vi "Serialize.vi"(8 "error in":errorcluster, 9 "OwningElement in":refnum<k20>, 10 "Document in":refnum<k20>, 11 "CustomDataType in":refnum<class "CustomData.lvclass">) -> (0 "error out":errorcluster, 1 "OwningElement out":refnum<k20>, 2 "Document out":refnum<k20>, 3 "CustomDataType out":refnum<class "CustomData.lvclass">)   [LabVIEW 2021, in "ProligentXMLGenerator.lvlib" / "CustomData.lvclass"]
uses:
  CustomData.lvclass
  CustomData.lvclass/CustomData.ctl
  Base/DOMSupport/DOMSupport.lvlib
  <vilib>/xml/NI_XML.lvlib
  <vilib>/xml/Close Reference(Node).vi
  CustomElement/CustomElement.lvclass
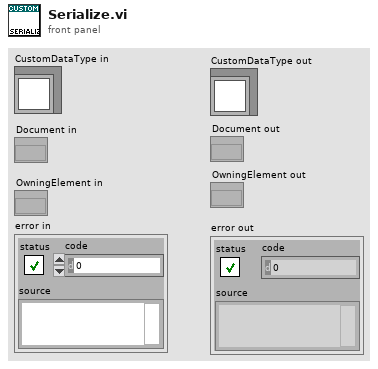
[diagram p1: front panel]
types:
  T1 = typedef "ProligentXMLGenerator.lvlib/CustomData.lvclass/Data.ctl" = cluster{"Name":string, "CustomElements":refnum<class "CustomElement.lvclass">[]}
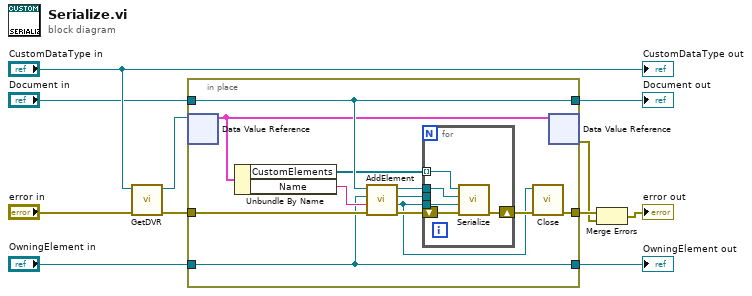
[diagram p0: block diagram]
diagram:
  n1 = call "GetDVR.vi"("error in"="error in", "CustomDataType"="CustomDataType in") -> ("error out"=w3:errorcluster, "DVRReference"=w2:refnum<data-value>)  [unwired: 8 in]
  n2 = in-place "In Place Element Structure" {
    in-place-border: [w21] -> w4
    in-place-border: "Document in" -> [w20]
    in-place-border: w3 -> [w23]
    in-place-border: "OwningElement in" -> [w19]
    in-place-border: [w20] -> w6
    in-place-border: [w19] -> w5
    n3 = in-place-dvr #1(w2) -> (w18:T1)  [unwired: 1 out]
    n4 = Unbundle By Name(w18) -> ("CustomElements"=w15:refnum<class "CustomElement.lvclass">[], "Name"=w22:string)
    n5 = call "AddElement.vi"("error in"=w23, "Name"=w22, "OwningElement in"=w19, "Document in"=w20) -> ("error out"=w17:errorcluster, "NewElement"=w13:refnum<k20>, "OwningElement out"=w14:refnum<k20>, "Document out"=w12:refnum<k20>)  [unwired: 4 in]
    n6 = for {
      shift-right: [w24] -> w16
      shift-left: w17 -> [w25]
      tunnel: w15 -> [w28] mode=indexing
      tunnel: w14 -> [_]
      tunnel: w13 -> [w27]
      tunnel: w12 -> [w26]
      n7 = call "Serialize.vi"("error in"=w25, "OwningElement in"=w27, "Document in"=w26, "CustomElement in"=w28) -> ("error out"=w24:errorcluster)  [unwired: 4 in, 3 out]
    }
    n8 = call-poly <vilib>:"Close.vi"("error in (no error)"=w16, "node"=w13) -> ("error out"=w21:errorcluster)  [unwired: 7 in]
    n9 = in-place-dvr #1(w18) -> (w1:errorcluster)  [unwired: 1 out]
  }
  "OwningElement out" <- w5
  "Document out" <- w6
  n10 = Merge Errors(w4, w1) -> (→"error out":errorcluster)
  "CustomDataType out" <- "CustomDataType in"
